vi "告警接口-告警存储-交互.vi"(10 "首次调用？":bool, 11 "筛选输入":T2={"componentParent"="氨氮", "equipVersion"="V2", "code"="0"}) -> (3 "data":T1)   [LabVIEW 2016, in "Alarm interface.lvlib"]
uses:
  Alarm interface.lvlib
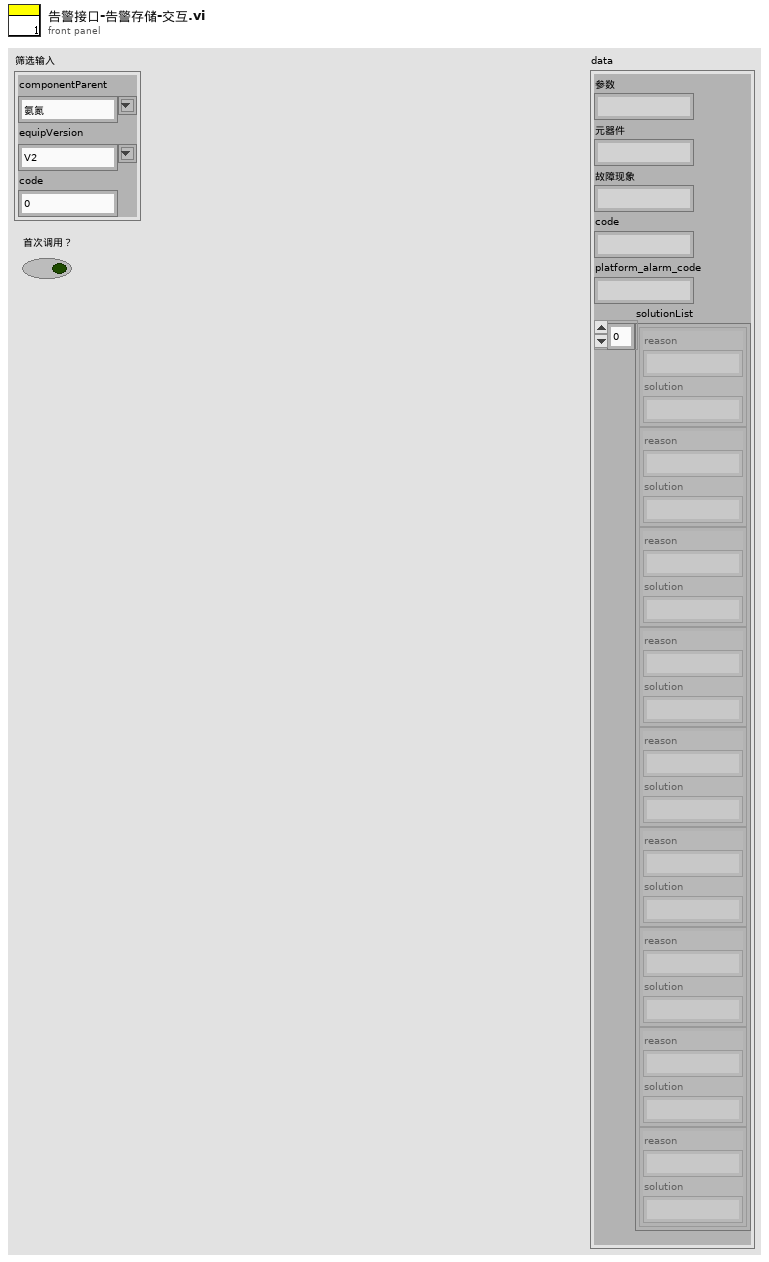
[diagram p1: front panel]
types:
  T1 = typedef "Alarm interface.lvlib/报警短信语音交互.ctl" = cluster{"参数":string, "元器件":string, "故障现象":string, "code":string, "platform_alarm_code":string, "solutionList":cluster{"reason":string, "solution":string}[]}
  T2 = cluster{"componentParent":string, "equipVersion":string, "code":string}
  T3 = typedef "报警信息字段定义.ctl" = cluster{"时间":timestamp, "参数":string, "元器件":string, "故障现象":string, "故障分析":string, "state":string, "code":string, "platform_alarm_code":string}
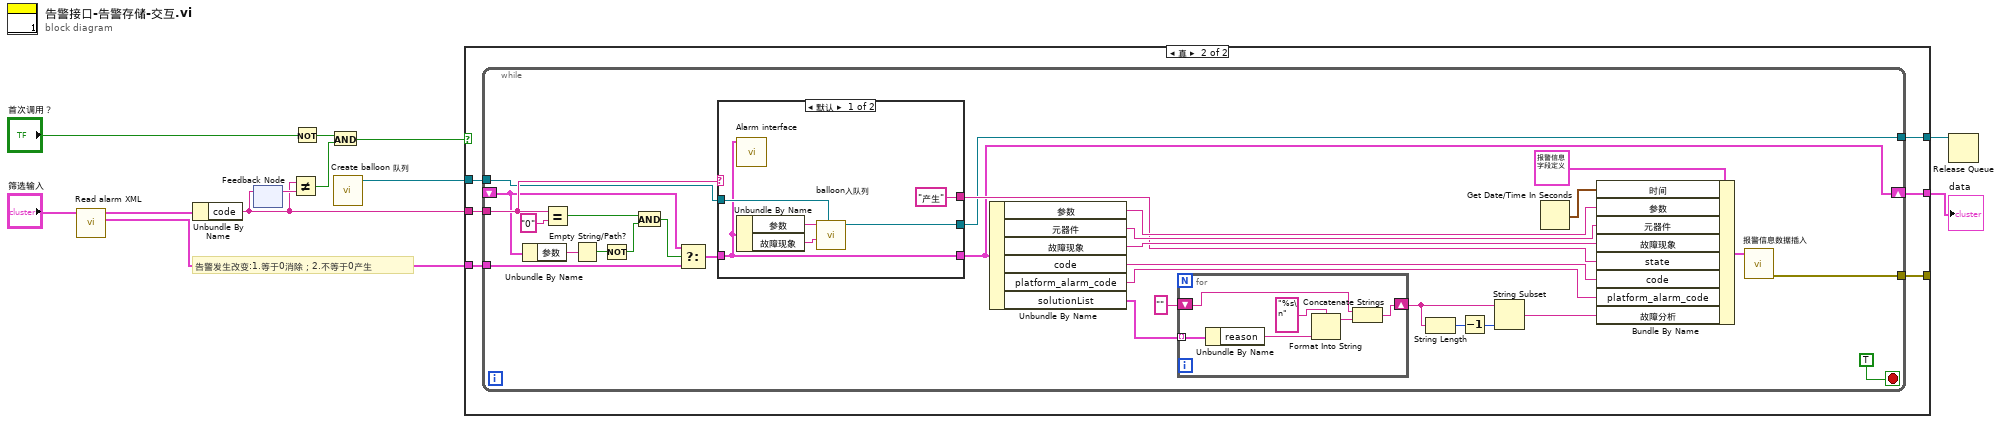
[diagram p0: block diagram]
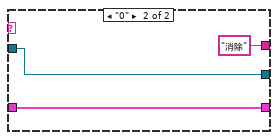
[diagram p3: hidden frame]
diagram:
  # "告警发生改变:1.等于0消除；2.不等于0产生"
  n1 = call "Read alarm XML.vi"("筛选输入"="筛选输入") -> ("筛选输出"=w10:T2, "data"=w8:T1)  [unwired: 8 in]
  n2 = Unbundle By Name(w10) -> ("code"=w9:string)
  n3 = feedback #1() -> (w11:string)  [unwired: 1 in]
  n4 = feedback-in #1(w9) -> ()
  n5 = Not Equal?(x=w9, y=w11) -> (x != y?=w7:bool)
  n6 = Not(x="首次调用？") -> (.not. x?=w5:bool)
  n7 = And(x=w5, y=w7) -> (x .and. y?=w4:bool)
  n8 = call "Create balloon 队列.vi"() -> ("队列输出"=w1:refnum<queue>)  [unwired: 11 in]
  n9 = case shown="真" w4 {
    tunnel: w9 -> [_ w20]
    tunnel: w8 -> [w14 w19]
    tunnel: [w14 w18] -> w2
    tunnel: w1 -> [w13 w17]
    tunnel: [w13 w16] -> w3
    tunnel: [_ w15] -> _
    frame False {
    }
    frame True {
      n10 = while {
        tunnel: w20 -> [w49]
        shift-right: [w30] -> w18
        shift-left: _ -> [w36]
        tunnel: w19 -> [w46]
        tunnel: w17 -> [w29]
        tunnel: [w28] -> w16
        tunnel: [w27] -> w15
        stop <- TRUE stop-if-true
        n11 = Unbundle By Name(w36) -> ("参数"=w35:string)
        n12 = Equal?(x=w49, y="0") -> (x = y?=w37:bool)
        n13 = Empty String/Path?(string/path=w35) -> (empty?=w34:bool)
        n14 = Not(x=w34) -> (.not. x?=w33:bool)
        n15 = And(x=w37, y=w33) -> (x .and. y?=w32:bool)
        n16 = Select(t=w36, s=w32, f=w46) -> (s? t:f=w47:T1)
        n17 = case shown="默认" w49 {
          tunnel: w47 -> [w57 w65]
          tunnel: [w57 w65] -> w30
          tunnel: ["产生" "消除"] -> w38
          tunnel: w29 -> [w59 w63]
          tunnel: [w58 w63] -> w28
          frame Default {
            n18 = call "Alarm interface.vi"("簇"=w57) -> ()  [unwired: 10 in, 1 out]
            n19 = Unbundle By Name(w57) -> ("参数"=w60:string, "故障现象"=w61:string)
            n20 = call "balloon入队列.vi"("队列"=w59, "告警信息"=w61, "参数名称"=w60) -> ("队列输出"=w58:refnum<queue>)  [unwired: 8 in]
          }
          frame "0" {
          }
        }
        n21 = Unbundle By Name(w30) -> ("参数"=w43:string, "元器件"=w42:string, "故障现象"=w41:string, "code"=w40:string, "platform_alarm_code"=w39:string, "solutionList"=w25:cluster{"reason":string, "solution":string}[])
        n22 = for {
          tunnel: w25 -> [w56] mode=indexing
          shift-right: [w51] -> w24
          shift-left: "" -> [w52]
          n23 = Unbundle By Name(w56) -> ("reason"=w54:string)
          n24 = Format Into String(format string="%s\n" ("格式字符串"), w54) -> (resulting string=w53:string)  [unwired: 2 in, 1 out]
          n25 = Concatenate Strings(w52, w53) -> (w51:string)
        }
        n26 = String Length(string=w24) -> (length=w23:i32)
        n27 = Decrement(x=w23) -> (x-1=w22:i32)
        n28 = String Subset(string=w24, length (rest)=w22) -> (substring=w21:string)  [unwired: 1 in]
        n29 = Get Date/Time In Seconds() -> (seconds since 1Jan1904=w44:timestamp)
        n30 = Bundle By Name(cluster=T3 {"时间"=timestamp(0 s since 1904-01-01), "参数"="", "元器件"="", "故障现象"="", "故障分析"="", "state"="", "code"="", "platform_alarm_code"=""} ("data"), "时间"=w44, "参数"=w43, "元器件"=w42, "故障现象"=w41, "state"=w38, "code"=w40, "platform_alarm_code"=w39, "故障分析"=w21) -> (w31:T3)
        n31 = call "报警信息数据插入.vi"("data"=w31) -> ("错误输出"=w27:errorcluster)  [unwired: 9 in]
      }
    }
  }
  "data" <- w2
  n32 = Release Queue(queue=w3) -> ()  [unwired: 2 in, 3 out]
